vi "RQST Comm Lookup Table_Actions.vi"(0 "ref in":T1, 5 "Connection In":T2, 7 "Index":i32, 9 "Method":T5, 11 "error in (no error)":errorcluster, 12 "Properties In":T4) -> (3 "All Properties":T4[](array[typedef]), 4 "ref out":T1, 6 "Connection Out":T2, 8 "All Connections":T2[](array[typedef]), 10 "Number of Connections":i32, 14 "Properties Out":T4, 15 "error out":errorcluster {"code" min=0 max=0})   [LabVIEW 2015, in "Diagnostics Addon Engine.lvlib"]
uses:
  Diagnostics Addon Engine.lvlib
  STM Lookup Table Ref.ctl
  Connection Manager/stm_TCPConnectionMethod.ctl
  TCP/stm_TCP Connection Info.ctl
  _SubVIs/stm_MetaDataElement.ctl
  Connection Manager/stm_TCPConnectionProperties.ctl
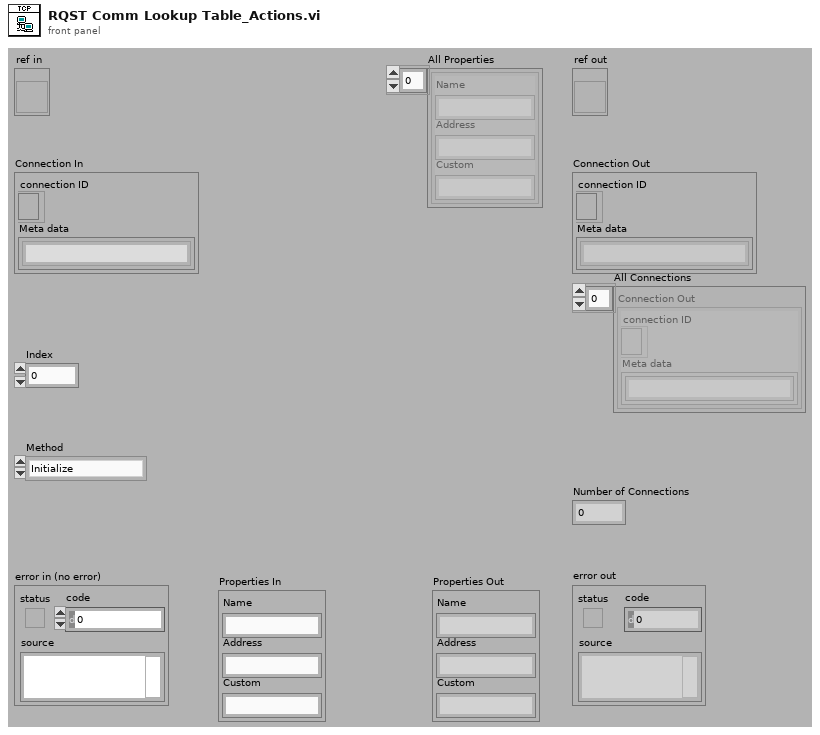
[diagram p1: front panel]
types:
  T1 = typedef "Diagnostics Addon Engine.lvlib/STM Lookup Table Ref.ctl" = refnum<vi>
  T2 = typedef "Diagnostics Addon Engine.lvlib/stm_TCP Connection Info.ctl" = cluster{"connection ID":refnum<k5>, "Meta data":T3[]}
  T3 = typedef "Diagnostics Addon Engine.lvlib/stm_MetaDataElement.ctl" = string
  T4 = typedef "Diagnostics Addon Engine.lvlib/stm_TCPConnectionProperties.ctl" = cluster{"Name":string, "Address":string, "Custom":string}
  T5 = typedef "Diagnostics Addon Engine.lvlib/stm_TCPConnectionMethod.ctl" = enum16{"Initialize", "Add Connection", "Set Properties", "Get Connection(s)", "Remove Connection", "Remove All Connections", "Get Connection Count"}
  T6 = typedef "stm_TCP Connection Info.ctl" = cluster{"connection ID":refnum<k5>, "Meta data":T7[]}
  T7 = typedef "stm_MetaDataElement.ctl" = string
  T8 = typedef "stm_TCPConnectionProperties.ctl" = cluster{"Name":string, "Address":string, "Custom":string}
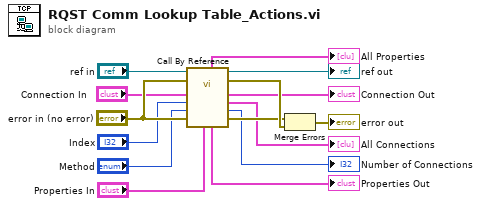
[diagram p0: block diagram]
diagram:
  n1 = call-by-ref "?"(reference="ref in", error in="error in (no error)", "Properties In"="Properties In", 8:"error in (no error)"="error in (no error)", "Method"="Method", "Index"="Index", "Connection In"="Connection In") -> (reference out=→"ref out":T1, error out=w14:errorcluster, 0:"error out"=w11:errorcluster, "Number of Connections"=→"Number of Connections":i32, "All Connections"=→"All Connections":T6[], "Connection Out"=→"Connection Out":T6, "Properties out"=→"Properties Out":T8, "All Properties"=→"All Properties":T8[])  [unwired: 1 in]
  n2 = Merge Errors(w11, w14) -> (→"error out":errorcluster)
